vi "FTW-NUM-EnumItems.vi"(7 "Enum":variant) -> (6 "Enum Items":string[](array[string]), 8 "Number of Items":i32, 10 "Selected Item":string)   [LabVIEW 2012]
panel:
  # "Inputs"
  # "Outputs"
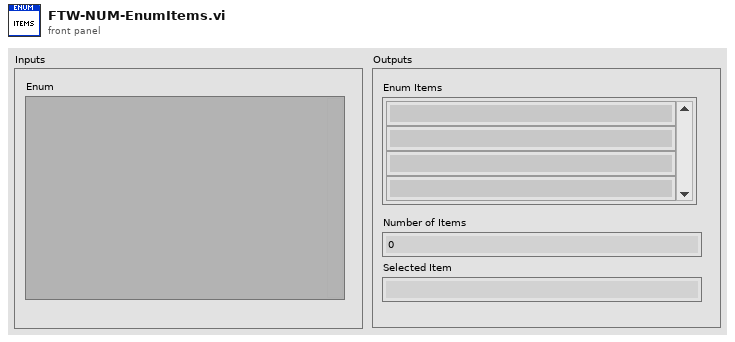
[diagram p1: front panel]
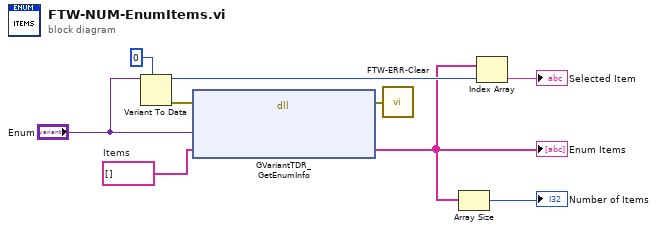
[diagram p0: block diagram]
diagram:
  w9 = string[] []  # Items
  n1 = Variant To Data(type=0, Variant="Enum") -> (data=w5:i32, error out=w6:errorcluster)  [unwired: 1 in]
  n2 = dll-call lib="LabVIEW" fn="GVariantTDR_GetEnumInfo"(error in=w6, "Input Enum Variant"="Enum", "Enum Items"=w9) -> (error out=w1:errorcluster, "Enum Items"=w3:string[])  [unwired: 4 in, 1 out]
  "Enum Items" <- w3
  n3 = call "FTW-ERR-Clear.vi"("error to snuff"=w1) -> ()  [unwired: 1 out]
  n4 = Array Size(array=w3) -> (size(s)=→"Number of Items":i32)
  n5 = Index Array(array=w3, index=w5) -> (element=→"Selected Item":string)
